vi "Config AO DC.vi"(6 "Channel config":T1, 8 "error in":errorcluster, 10 "Voltage":dbl=1.0 caption="Amplitude", 11 "task in":refnum<k21>) -> (0 "error out":errorcluster, 3 "task out":refnum<k21>)   [LabVIEW 2019]
doc: "This example demonstrates how to acquire a continuous amount of data (Waveform) using the DAQ device's internal clock. It also shows how to synchronize two devices for different device families (E Series, S Series, M Series, X Series, DSA, and SC Express), to simultaneously acquire the data.\n\nFor instructions on how to connect your signals to the DAQ device, refer to your device documentation."
uses:
  <vilib>/DAQmx/create/channels.llb/DAQmx Create Channel (AO-Voltage-Basic).vi
  <vilib>/DAQmx/miscellaneous.llb/DAQmx Fill In Error Info.vi
panel:
  # "Config AO - DC"
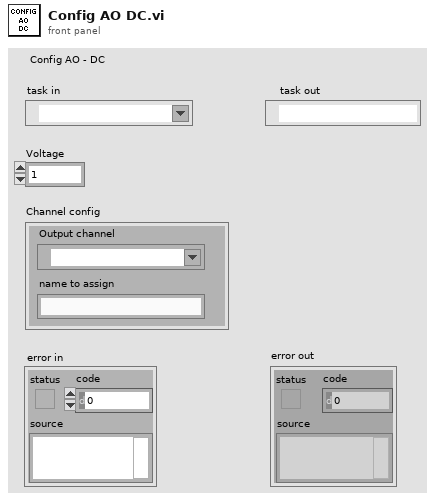
[diagram p1: front panel]
types:
  T1 = cluster{"Output channel":tag, "name to assign":string}
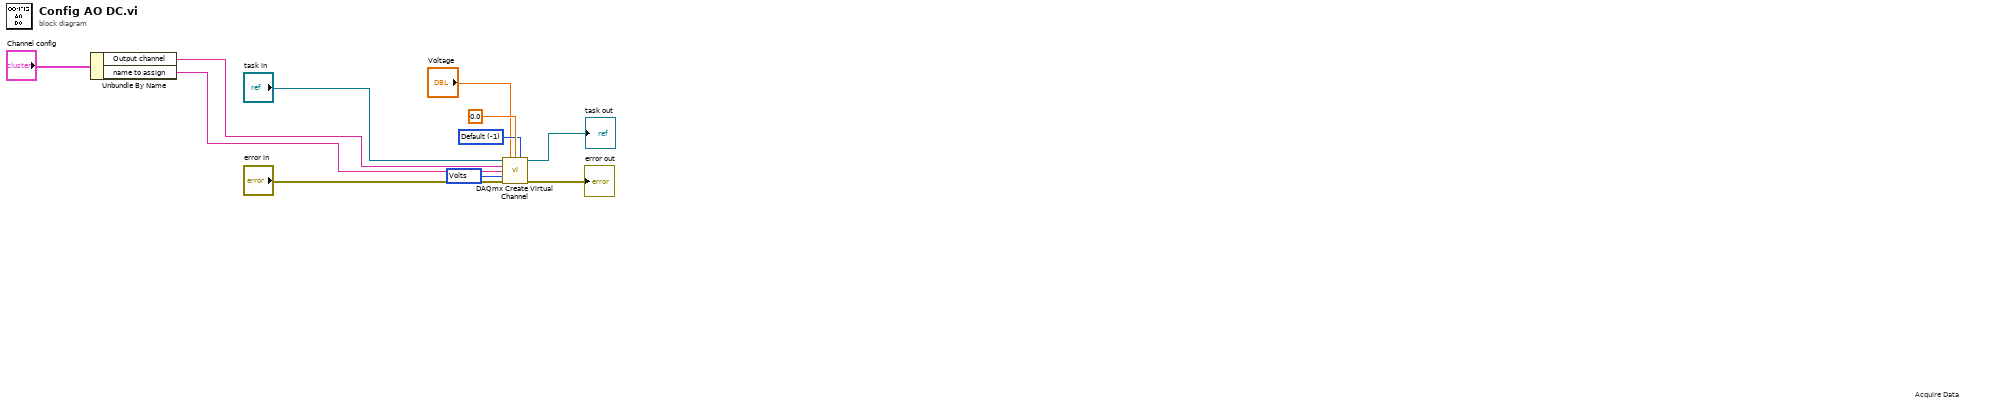
[diagram p0: block diagram]
diagram:
  w4 = 10348 items=["Volts"=10348, "From Custom Scale"=10065] ("units")
  w5 = -1 items=["Default"=-1, "RSE"=10083, "Differential"=10106, "Pseudodifferential"=12529] ("output terminal configuration")
  # "Acquire Data"
  n1 = Unbundle By Name("Channel config") -> ("Output channel"=w7:tag, "name to assign"=w6:string)
  n2 = call-poly <vilib>:"DAQmx Create Virtual Channel.vi"("task in"="task in", "maximum value"="Voltage", "minimum value"=0.0, "output terminal configuration"=w5, "physical channels"=w7, "name to assign"=w6, "units"=w4, "error in"="error in") -> ("task out"=→"task out":refnum<k21>, "error out"=→"error out":errorcluster)  [unwired: 6 in]
